vi "Grenzwertberechnung.vi"(11 "Durchfluss":sgl) -> (3 "Grenze":sgl format="%#.10f")   [LabVIEW 2020, in "EPA 1065.lvlib" / "Dichtheitstest 1065-345.lvlib"]
uses:
  Dichtheitstest 1065-345.lvlib
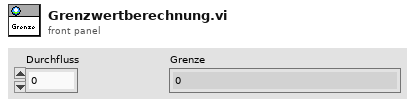
[diagram p1: front panel]
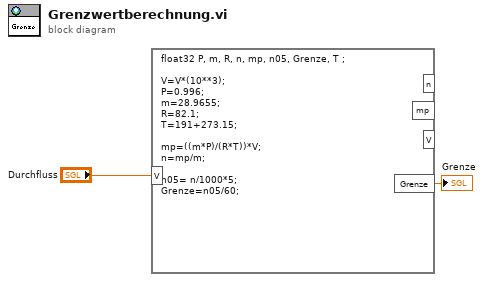
[diagram p0: block diagram]
diagram:
  n1 = formula code="float32 P, m, R, n, mp, n05, Grenze, T ;\n\nV=V*(10**3);\nP=0.996;\nm=28.9655;\nR=82.1;\nT=191+273.15;\n\nmp=((m*P)/(R*T))*V;\nn=mp/m;\n\nn05= n/1000*5;\nGrenze=n05/60;"("V"="Durchfluss") -> ("Grenze"=→"Grenze":sgl)  [unwired: 3 out]
